vi "Setup XNode Detailed Help.vi"(1 "Terms":T10, 2 "Bounds":T13, 3 "Image":T2) -> (0 "Detailed Help Info":T1)   [LabVIEW 2025, in "XNode Support.lvlib"]
uses:
  XNode Support.lvlib
  <vilib>/XNodeSupport/XNodeImage.ctl
  <vilib>/XNodeSupport/XNodeBounds.ctl
  <vilib>/XNodeSupport/XNodeInt.ctl
  <vilib>/XNodeSupport/XNodeTerm4Array.ctl
  <vilib>/XNodeSupport/XNodeTerm4.ctl
  <vilib>/XNodeSupport/XNodeString.ctl
  <vilib>/XNodeSupport/XNodeVariant.ctl
  <vilib>/XNodeSupport/XNodeRect32.ctl
  <vilib>/XNodeSupport/XNodeBool.ctl
  <vilib>/XNodeSupport/XNodeTermDirection.ctl
  <vilib>/XNodeSupport/XNodeDetailedHelpInfo.ctl
  <vilib>/XNodeSupport/XNodeTerms.ctl
  <vilib>/XNodeSupport/XNodeTerm.ctl
  <vilib>/XNodeSupport/NI_XNodeSupport.lvlib
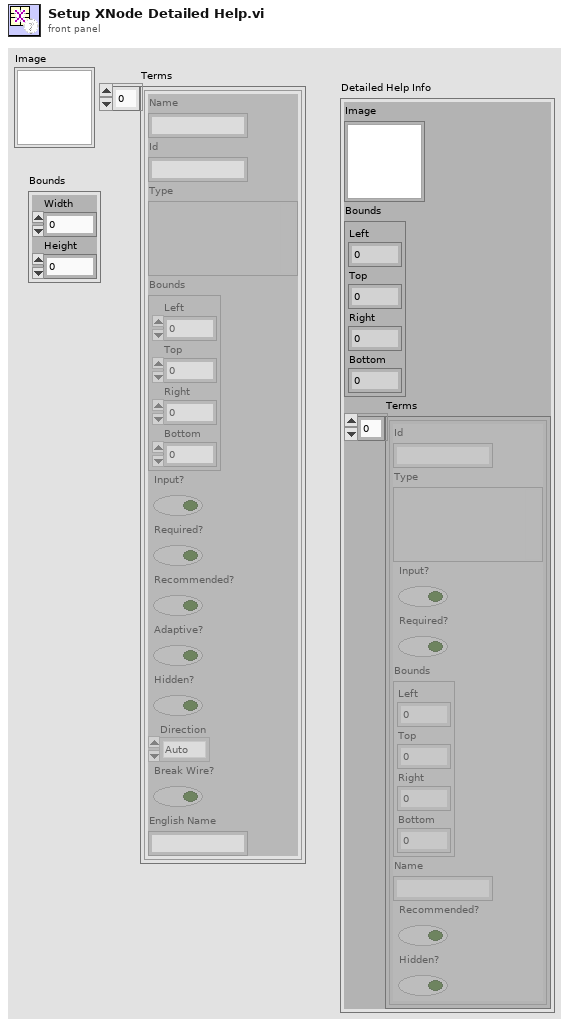
[diagram p1: front panel]
types:
  T1 = typedef "NI_XNodeSupport.lvlib/XNodeDetailedHelpInfo.ctl" = cluster{"Image":T2, "Bounds":T3, "Terms":T5}
  T2 = typedef "NI_XNodeSupport.lvlib/XNodeImage.ctl" = picture
  T3 = typedef "NI_XNodeSupport.lvlib/XNodeRect32.ctl" = cluster{"Left":T4, "Top":T4, "Right":T4, "Bottom":T4}
  T4 = typedef "NI_XNodeSupport.lvlib/XNodeInt.ctl" = i32
  T5 = typedef "NI_XNodeSupport.lvlib/XNodeTerms.ctl" = T6[]
  T6 = typedef "NI_XNodeSupport.lvlib/XNodeTerm.ctl" = cluster{"Id":T7, "Type":T8, "Input?":T9, "Required?":T9, "Bounds":T3, "Name":T7, "Recommended?":T9, "Hidden?":T9}
  T7 = typedef "NI_XNodeSupport.lvlib/XNodeString.ctl" = string
  T8 = typedef "NI_XNodeSupport.lvlib/XNodeVariant.ctl" = variant
  T9 = typedef "NI_XNodeSupport.lvlib/XNodeBool.ctl" = bool
  T10 = typedef "NI_XNodeSupport.lvlib/XNodeTerm4Array.ctl" = T11[]
  T11 = typedef "NI_XNodeSupport.lvlib/XNodeTerm4.ctl" = cluster{"Name":T7, "Id":T7, "Type":T8, "Bounds":T3, "Input?":T9, "Required?":T9, "Recommended?":T9, "Adaptive?":T9, "Hidden?":T9, "Direction":T12, "Break Wire?":T9, "English Name":T7}
  T12 = typedef "NI_XNodeSupport.lvlib/XNodeTermDirection.ctl" = enum32{"Auto", "Up", "Down", "Left", "Right", "Center"}
  T13 = typedef "NI_XNodeSupport.lvlib/XNodeBounds.ctl" = cluster{"Width":T4, "Height":T4}
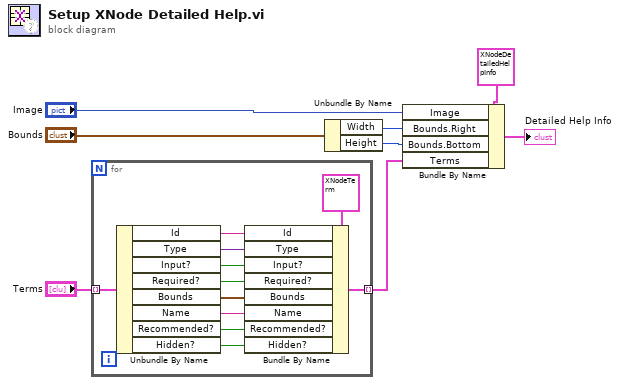
[diagram p0: block diagram]
diagram:
  n1 = for {
    tunnel: "Terms" -> [w19] mode=indexing
    tunnel: [w10] -> w4 mode=indexing
    n2 = Unbundle By Name(w19) -> ("Id"=w18:T7, "Type"=w17:T8, "Input?"=w16:T9, "Required?"=w15:T9, "Bounds"=w14:T3, "Name"=w13:T7, "Recommended?"=w12:T9, "Hidden?"=w11:T9)
    n3 = Bundle By Name(cluster=T6 {"Id"="", "Type"=variant, "Input?"=FALSE, "Required?"=FALSE, "Bounds"={"Left"=0, "Top"=0, "Right"=0, "Bottom"=0}, "Name"="", "Recommended?"=FALSE, "Hidden?"=FALSE} ("Term"), "Id"=w18, "Type"=w17, "Input?"=w16, "Required?"=w15, "Bounds"=w14, "Name"=w13, "Recommended?"=w12, "Hidden?"=w11) -> (w10:T6)
  }
  n4 = Unbundle By Name("Bounds") -> ("Width"=w8:T4, "Height"=w7:T4)
  n5 = Bundle By Name(cluster=T1 {"Image"=bytes[0], "Bounds"={"Left"=0, "Top"=0, "Right"=0, "Bottom"=0}, "Terms"=[]} ("Detailed Help Info"), "Image"="Image", "Bounds.Right"=w8, "Bounds.Bottom"=w7, "Terms"=w4) -> (→"Detailed Help Info":T1)
